vi "FTW-Container-Value-Integer.vi"(0 "JSON":refnum<class "FTW-Container.lvclass">, 11 "error in":errorcluster) -> (4 "JSON out":refnum<class "FTW-Container.lvclass">, 8 "Value":i64, 15 "error out":errorcluster)   [LabVIEW 2015, in "FTW-Container.lvclass"]
uses:
  FTW-Container.lvclass
  FTW-Container.lvclass/FTW-Container.ctl
  <vilib>/Utility/Data Type/NI_Data Type.lvlib
panel:
  # "Inputs"
  # "Outputs"
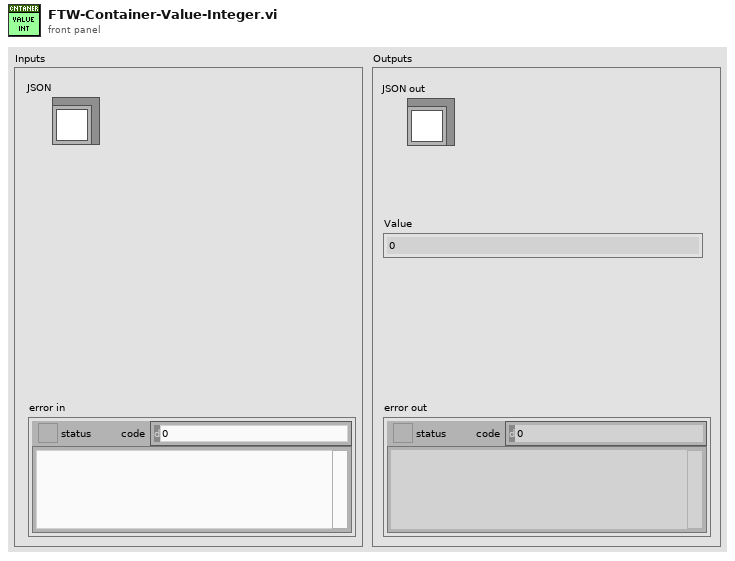
[diagram p1: front panel]
types:
  T1 = typedef "NI_Data Type.lvlib/Data Type.ctl" = enum8{"Invalid Type", "Void", "I8", "I16", "I32", "I64", "U8", "U16", "U32", "U64", "Single Float", "Double Float", "Extended Float", "Single Complex", "Double Complex", "Extended Complex", "Enum U8", "Enum U16", "Enum U32", "Enum U64", "Single Float With Unit", "Double Float With Unit", "Extended Float With Unit", "Single Complex with Unit", "Double Complex with Unit", "Extended Complex with Unit", "Boolean", "String", "Path", "Picture", "Tag", "Array", "Cluster", "Variant", "LV Variant", "Waveform", "Timestamp", "Digital Waveform", "Digital Data", "ExpressData", "Refnum", "External Data", "VI", "Poly VI", "LabVIEW Class Instance", "Fixed Point"}
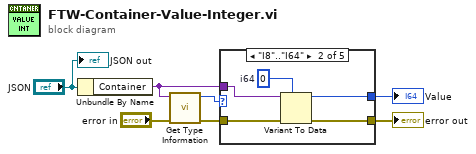
[diagram p0: block diagram]
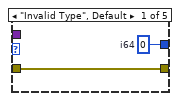
[diagram p2: hidden frame]
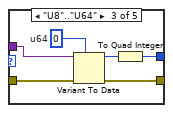
[diagram p3: hidden frame]
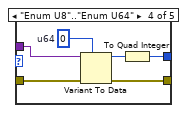
[diagram p4: hidden frame]
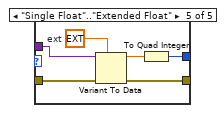
[diagram p5: hidden frame]
diagram:
  n1 = Unbundle By Name("JSON") -> ("Container"=w1:variant)
  n2 = call <vilib>:"Get Type Information.vi"("error in (no error)"="error in", "Variant"=w1) -> ("error out"=w7:errorcluster, "Type"=w6:T1)  [unwired: 5 in, 3 out]
  n3 = case shown="\"I8\"..\"I64\"" w6 {
    tunnel: w7 -> [w9 w13 w19 w25 w31]
    tunnel: w1 -> [_ w12 w18 w24 w30]
    tunnel: [w9 w11 w17 w23 w29] -> w4
    tunnel: [w8 w10 w15 w21 w27] -> w3
    frame "Invalid Type", Default {
      w8 = i64 0  # i64
    }
    frame "I8".."I64" {
      w14 = i64 0  # i64
      n4 = Variant To Data(error in=w13, type=w14, Variant=w12) -> (data=w10:i64, error out=w11:errorcluster)
    }
    frame "U8".."U64" {
      w20 = u64 0  # u64
      n5 = Variant To Data(error in=w19, type=w20, Variant=w18) -> (data=w16:u64, error out=w17:errorcluster)
      n6 = To Quad Integer(1:w16) -> (0:w15:i64)
    }
    frame "Enum U8".."Enum U64" {
      w26 = u64 0  # u64
      n7 = Variant To Data(error in=w25, type=w26, Variant=w24) -> (data=w22:u64, error out=w23:errorcluster)
      n8 = To Quad Integer(1:w22) -> (0:w21:i64)
    }
    frame "Single Float".."Extended Float" {
      w32 = ext 0.0  # ext
      n9 = Variant To Data(error in=w31, type=w32, Variant=w30) -> (data=w28:ext, error out=w29:errorcluster)
      n10 = To Quad Integer(1:w28) -> (0:w27:i64)
    }
  }
  "error out" <- w4
  "Value" <- w3
  "JSON out" <- "JSON"
